vi "Vision Processing.vi"(4 "error in (no error)":errorcluster, 7 "Image Size":T1=enum."320x240") -> ()   [LabVIEW 2017]
doc: "This VI runs in parallel to other tasks. It gets images from the camera, processes them for color or shape and use that information to affect robot behavior."
uses:
  <vilib>/Rock Robotics/WPI/Camera/WPI_CameraImageSize.ctl
  <vilib>/Rock Robotics/WPI/Camera/WPI_CameraWhite Balance Values.ctl
  <vilib>/Rock Robotics/WPI/Camera/WPI_CameraExposure Values.ctl
  <vilib>/Rock Robotics/WPI/Camera/WPI_CameraFrameRate.ctl
  Robot Global Data.vi
panel:
  in  "Image Size 2":T1=enum."320x240"
  in  "error in (no error) 2":errorcluster
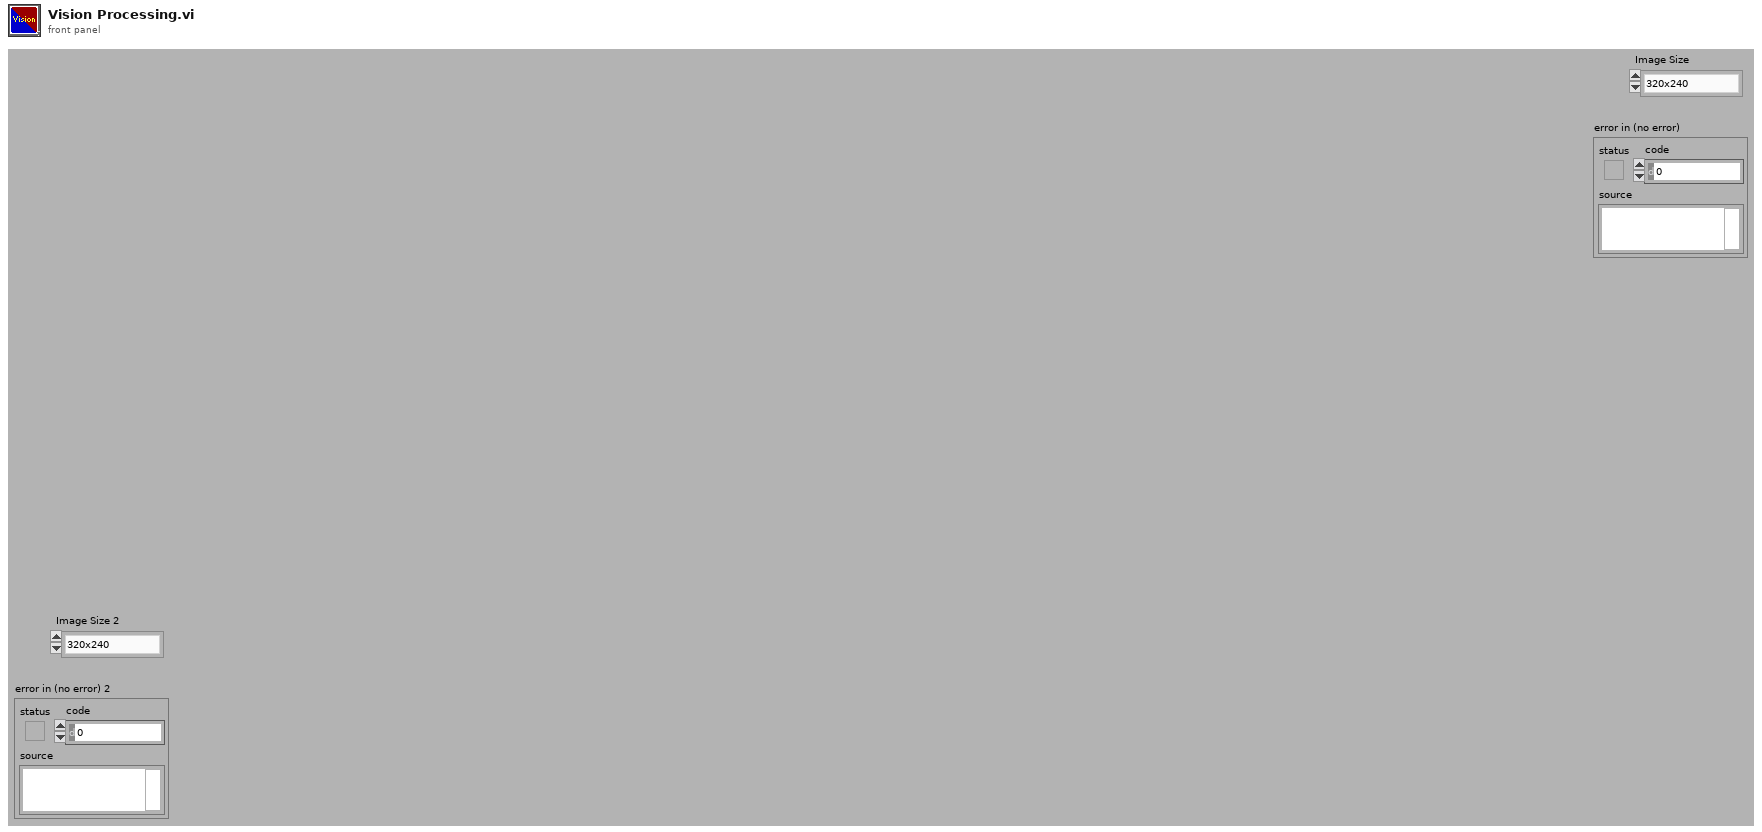
[diagram p1: front panel]
types:
  T1 = typedef "WPI_CameraImageSize.ctl" = enum16{"640x480", "320x240", "160x120", "Custom"}
  T2 = typedef "WPI_CameraFrameRate.ctl" = u32
  T3 = typedef "WPI_CameraExposure Values.ctl" = enum16{"Auto", "Flicker-free 50 Hz", "Flicker-free 60 Hz", "Hold current", "Custom"}
  T4 = typedef "WPI_CameraWhite Balance Values.ctl" = enum16{"Auto", "Fixed indoor", "Fixed outdoor 1", "Fixed outdoor 2", "Fixed fluorescent 1", "Fixed fluorescent 2", "Hold current", "Custom"}
  T5 = typedef "Image Type" = u32
  T6 = typedef "WPI_CameraDevRef.ctl" = cluster{"Camera Address":string, "CameraStatus":errorcluster}
  T7 = typedef "IMAQ Image.ctl" = refnum<image>
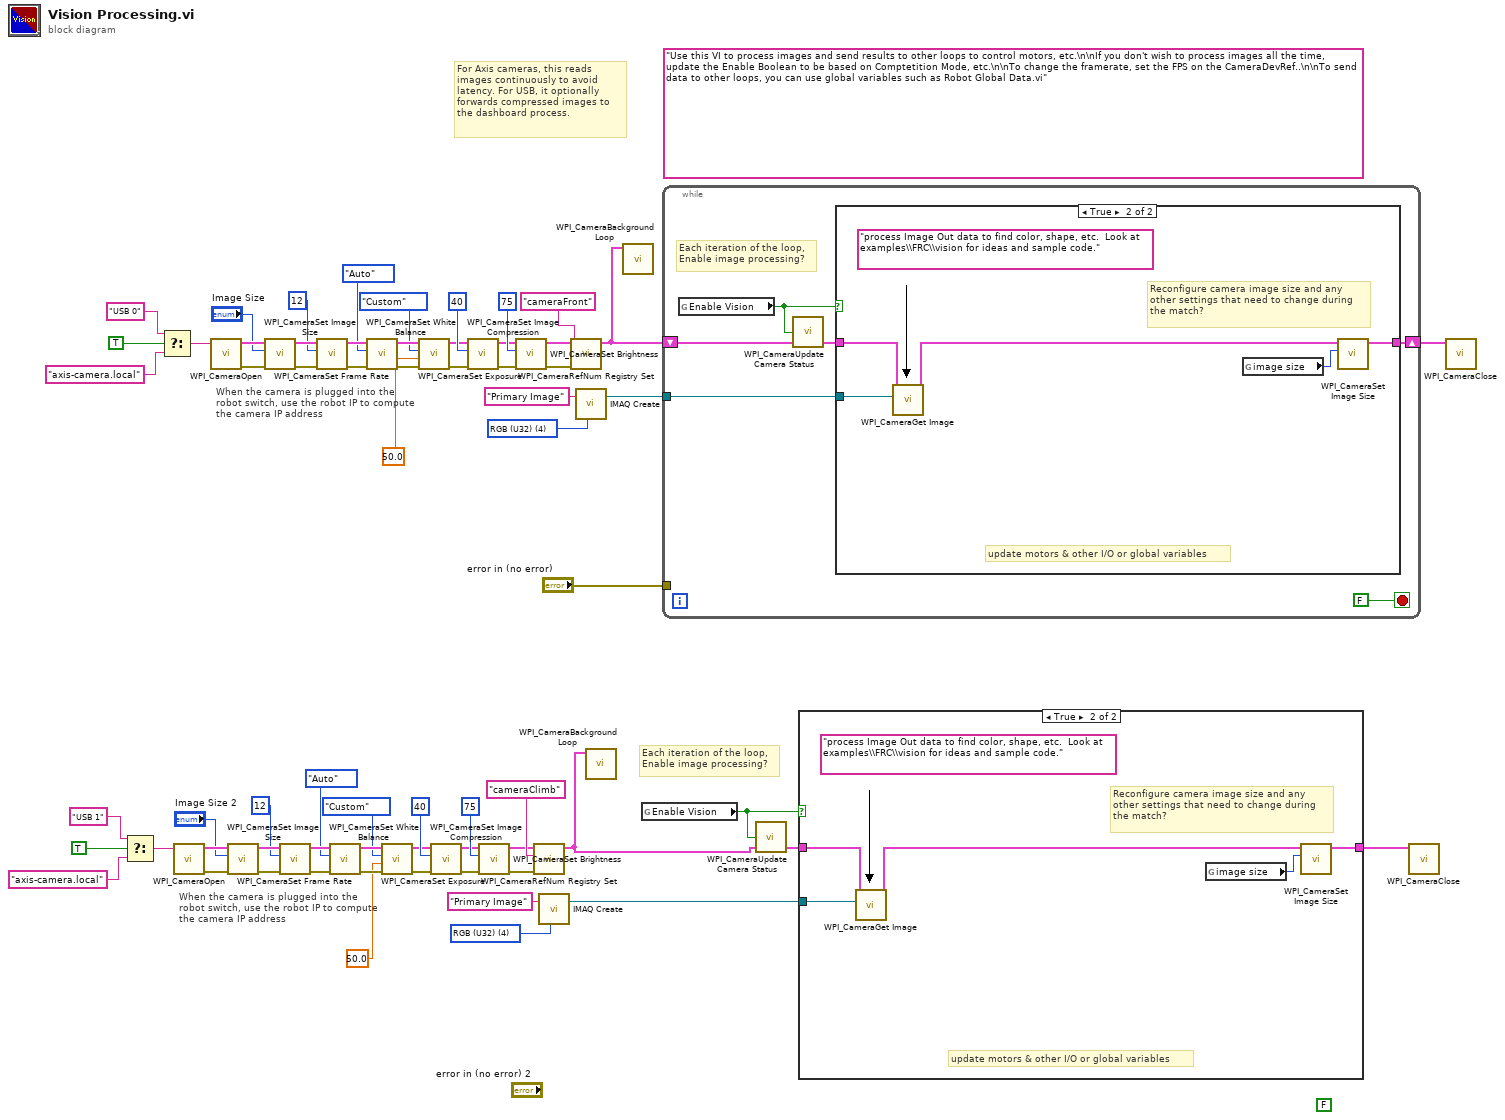
[diagram p0: block diagram]
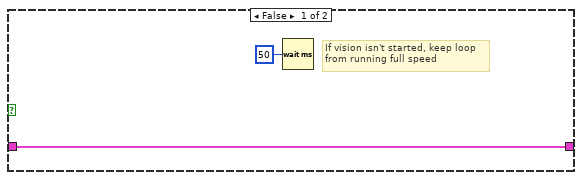
[diagram p2: hidden frame]
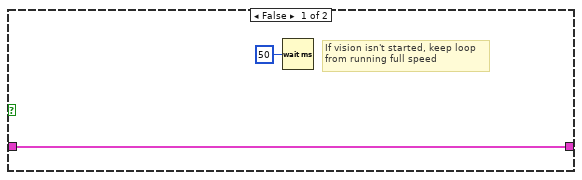
[diagram p3: hidden frame]
diagram:
  w34 = T5 4 items=["Grayscale (U8)", "Grayscale (I16)", "Grayscale (SGL)", "Complex (CSG)", "RGB (U32)", "HSL (U32)", "RGB (U64)"] ("Image Type")
  (unwired) FALSE
  (unwired) "Use this VI to process images and send results to other loops to control motors, etc.\n\nIf you don't wish to process images all the time, update the Enable Boolean to be based on Comptetition Mode, etc.\n\nTo change the framerate, set the FPS on the CameraDevRef..\n\nTo send data to other loops, you can use global variables such as Robot Global Data.vi"
  w65 = T5 4 items=["Grayscale (U8)", "Grayscale (I16)", "Grayscale (SGL)", "Complex (CSG)", "RGB (U32)", "HSL (U32)", "RGB (U64)"] ("Image Type")
  # "When the camera is plugged into the\nrobot switch, use the robot IP to compute\nthe camera IP address"
  # "Each iteration of the loop,\nEnable image processing?"
  # "When the camera is plugged into the\nrobot switch, use the robot IP to compute\nthe camera IP address"
  # "For Axis cameras, this reads\nimages continuously to avoid\nlatency. For USB, it optionally\nforwards compressed images to\nthe dashboard process."
  n1 = Select(t="USB 1" ("format string"), s=TRUE ("dot notation? (F)"), f="axis-camera.local" ("format string")) -> (s? t:f=w9:string)
  n2 = Select(t="USB 0" ("format string"), s=TRUE ("dot notation? (F)"), f="axis-camera.local" ("format string")) -> (s? t:f=w36:string)
  n3 = call <vilib>:"WPI_CameraOpen.vi"("Camera Address"=w9) -> ("error out"=w23:errorcluster, "CameraDevRef"=w24:T6)  [unwired: 1 in, 8 out]
  n4 = call <vilib>:"WPI_CameraOpen.vi"("Camera Address"=w36) -> ("error out"=w53:errorcluster, "CameraDevRef"=w54:T6)  [unwired: 1 in, 8 out]
  n5 = call <vilib>:"WPI_CameraSet Image Size.vi"("error in (no error)"=w23, "Image Size"="Image Size 2", "CameraDevRef"=w24) -> ("error out"=w22:errorcluster, "CameraDevRef Out"=w25:T6)  [unwired: 1 in, 6 out]
  n6 = call <vilib>:"WPI_CameraSet Image Size.vi"("error in (no error)"=w53, "Image Size"="Image Size", "CameraDevRef"=w54) -> ("error out"=w52:errorcluster, "CameraDevRef Out"=w55:T6)  [unwired: 1 in, 6 out]
  n7 = call <vilib>:"WPI_CameraSet Frame Rate.vi"("error in (no error)"=w22, "Frame Rate (fps)"=T2 12, "CameraDevRef"=w25) -> ("error out"=w21:errorcluster, "CameraDevRef Out"=w27:T6)  [unwired: 7 out]
  n8 = call <vilib>:"WPI_CameraSet Frame Rate.vi"("error in (no error)"=w52, "Frame Rate (fps)"=T2 12, "CameraDevRef"=w55) -> ("error out"=w51:errorcluster, "CameraDevRef Out"=w57:T6)  [unwired: 7 out]
  n9 = call <vilib>:"WPI_CameraSet White Balance.vi"("error in (no error)"=w21, "White Balance"=WPI_CameraWhite_Balance_Values."Auto", "CameraDevRef"=w27) -> ("error out"=w20:errorcluster, "CameraDevRef Out"=w26:T6)  [unwired: 1 in, 6 out]
  n10 = call <vilib>:"WPI_CameraSet White Balance.vi"("error in (no error)"=w51, "White Balance"=WPI_CameraWhite_Balance_Values."Auto", "CameraDevRef"=w57) -> ("error out"=w50:errorcluster, "CameraDevRef Out"=w56:T6)  [unwired: 1 in, 6 out]
  n11 = call <vilib>:"WPI_CameraSet Exposure.vi"("error in (no error)"=w20, "Exposure (%)"=50.0, "Exposure"=WPI_CameraExposure_Values."Custom", "CameraDevRef"=w26) -> ("error out"=w19:errorcluster, "CameraDevRef Out"=w29:T6)  [unwired: 6 out]
  n12 = call <vilib>:"WPI_CameraSet Exposure.vi"("error in (no error)"=w50, "Exposure (%)"=50.0, "Exposure"=WPI_CameraExposure_Values."Custom", "CameraDevRef"=w56) -> ("error out"=w49:errorcluster, "CameraDevRef Out"=w59:T6)  [unwired: 6 out]
  n13 = call <vilib>:"WPI_CameraSet Image Compression.vi"("error in (no error)"=w19, "Compression"=40, "CameraDevRef"=w29) -> ("error out"=w18:errorcluster, "CameraDevRef Out"=w28:T6)  [unwired: 7 out]
  n14 = call <vilib>:"WPI_CameraSet Image Compression.vi"("error in (no error)"=w49, "Compression"=40, "CameraDevRef"=w59) -> ("error out"=w48:errorcluster, "CameraDevRef Out"=w58:T6)  [unwired: 7 out]
  n15 = call <vilib>:"WPI_CameraSet Brightness.vi"("error in (no error)"=w18, "Brightness"=75, "CameraDevRef"=w28) -> ("error out"=w16:errorcluster, "CameraDevRef Out"=w17:T6)  [unwired: 1 in, 6 out]
  n16 = call <vilib>:"WPI_CameraSet Brightness.vi"("error in (no error)"=w48, "Brightness"=75, "CameraDevRef"=w58) -> ("error out"=w46:errorcluster, "CameraDevRef Out"=w47:T6)  [unwired: 1 in, 6 out]
  n17 = call <vilib>:"WPI_CameraRefNum Registry Set.vi"("error in (no error)"=w16, "refnum name"="cameraClimb", "CameraDevRef"=w17) -> ("CameraDevRef"=w4:T6)  [unwired: 1 in, 7 out]
  n18 = call "IMAQ Create"("Image Name"="Primary Image", "Image Type"=w34) -> ("New Image"=w5:T7)  [unwired: 2 in, 2 out]
  n19 = call <vilib>:"WPI_CameraRefNum Registry Set.vi"("error in (no error)"=w46, "refnum name"="cameraFront", "CameraDevRef"=w47) -> ("CameraDevRef"=w42:T6)  [unwired: 1 in, 7 out]
  n20 = call "IMAQ Create"("Image Name"="Primary Image", "Image Type"=w65) -> ("New Image"=w63:T7)  [unwired: 2 in, 2 out]
  n21 = call <vilib>:"WPI_CameraBackground Loop.vi"("CameraDevRef"=w4) -> ()  [unwired: 11 in]
  n22 = call <vilib>:"WPI_CameraBackground Loop.vi"("CameraDevRef"=w42) -> ()  [unwired: 11 in]
  n23 = global read "Robot Global Data.vi" "Enable Vision"() -> (w6:bool)
  n24 = while {
    shift-right: [w70] -> w40
    shift-left: w42 -> [w68]
    tunnel: w63 -> [w69]
    tunnel: "error in (no error)" -> [_]
    stop <- FALSE stop-if-true
    # "Each iteration of the loop,\nEnable image processing?"
    n25 = global read "Robot Global Data.vi" "Enable Vision"() -> (w66:bool)
    n26 = call <vilib>:"WPI_CameraUpdate Camera Status.vi"("CameraDevRef In"=w68, "Enable Vision"=w66) -> ("CameraDevRef Out"=w67:T6)  [unwired: 3 in]
    n27 = case shown="True" w66 {
      tunnel: w69 -> [_ w77]
      tunnel: [w73 w78] -> w70
      tunnel: w67 -> [w73 w75]
      frame False {
        # "If vision isn't started, keep loop\nfrom running full speed"
        n28 = Wait (ms)(milliseconds to wait=u32 50) -> ()  [unwired: 1 out]
      }
      frame True {
        (unwired) "process Image Out data to find color, shape, etc.  Look at examples\\FRC\\vision for ideas and sample code."
        # "update motors & other I/O or global variables"
        # "Reconfigure camera image size and any\nother settings that need to change during\nthe match?"
        n29 = call <vilib>:"WPI_CameraGet Image.vi"("Image"=w77, "CameraDevRef"=w75) -> ("CameraDevRef Out"=w74:T6)  [unwired: 1 in, 8 out]
        n30 = global read "Robot Global Data.vi" "image size"() -> (w76:T1)
        n31 = call <vilib>:"WPI_CameraSet Image Size.vi"("Image Size"=w76, "CameraDevRef"=w74) -> ("CameraDevRef Out"=w78:T6)  [unwired: 2 in, 7 out]
      }
    }
  }
  n32 = call <vilib>:"WPI_CameraUpdate Camera Status.vi"("CameraDevRef In"=w4, "Enable Vision"=w6) -> ("CameraDevRef Out"=w7:T6)  [unwired: 3 in]
  n33 = case shown="True" w6 {
    tunnel: [w80 w85] -> w1
    tunnel: w7 -> [w80 w83]
    tunnel: w5 -> [_ w81]
    frame False {
      # "If vision isn't started, keep loop\nfrom running full speed"
      n34 = Wait (ms)(milliseconds to wait=u32 50) -> ()  [unwired: 1 out]
    }
    frame True {
      (unwired) "process Image Out data to find color, shape, etc.  Look at examples\\FRC\\vision for ideas and sample code."
      # "update motors & other I/O or global variables"
      # "Reconfigure camera image size and any\nother settings that need to change during\nthe match?"
      n35 = call <vilib>:"WPI_CameraGet Image.vi"("Image"=w81, "CameraDevRef"=w83) -> ("CameraDevRef Out"=w82:T6)  [unwired: 1 in, 8 out]
      n36 = global read "Robot Global Data.vi" "image size"() -> (w84:T1)
      n37 = call <vilib>:"WPI_CameraSet Image Size.vi"("Image Size"=w84, "CameraDevRef"=w82) -> ("CameraDevRef Out"=w85:T6)  [unwired: 2 in, 7 out]
    }
  }
  n38 = call <vilib>:"WPI_CameraClose.vi"("CameraDevRef"=w1) -> ()  [unwired: 1 in, 10 out]
  n39 = call <vilib>:"WPI_CameraClose.vi"("CameraDevRef"=w40) -> ()  [unwired: 1 in, 10 out]
